vi "DAQ_daqmx.vi"() -> ()   [LabVIEW 2020]
uses:
  <vilib>/Utility/error.llb/DialogType.ctl
  <vilib>/Utility/sysdir.llb/System Directory Type.ctl
  <vilib>/DAQmx/read.llb/DAQmx Read (Analog 2D DBL NChan NSamp).vi
  <vilib>/DAQmx/create/channels.llb/DAQmx Create Channel (AI-Voltage-Basic).vi
  <vilib>/DAQmx/configure/timing.llb/DAQmx Timing (Sample Clock).vi
  <vilib>/DAQmx/configure/trigger.llb/DAQmx Start Trigger (None).vi
  <vilib>/DAQmx/miscellaneous.llb/DAQmx Fill In Error Info.vi
panel:
  in  "Save Button":bool
  out "Waveform Chart 2":dbl[][](graph)
  out "data":dbl[][](array[numeric]) format="%0.2f"
  in  "stop":bool
  out "Waveform Chart":dbl[][](graph)
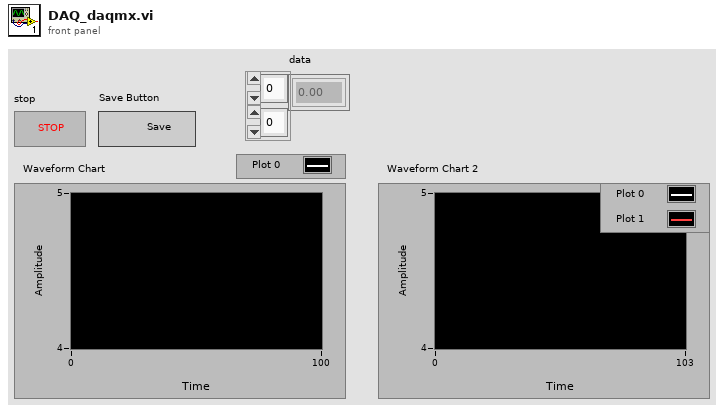
[diagram p1: front panel]
types:
  T1 = typedef "DialogType.ctl" = u16
  T2 = typedef "System Directory Type.ctl" = i32
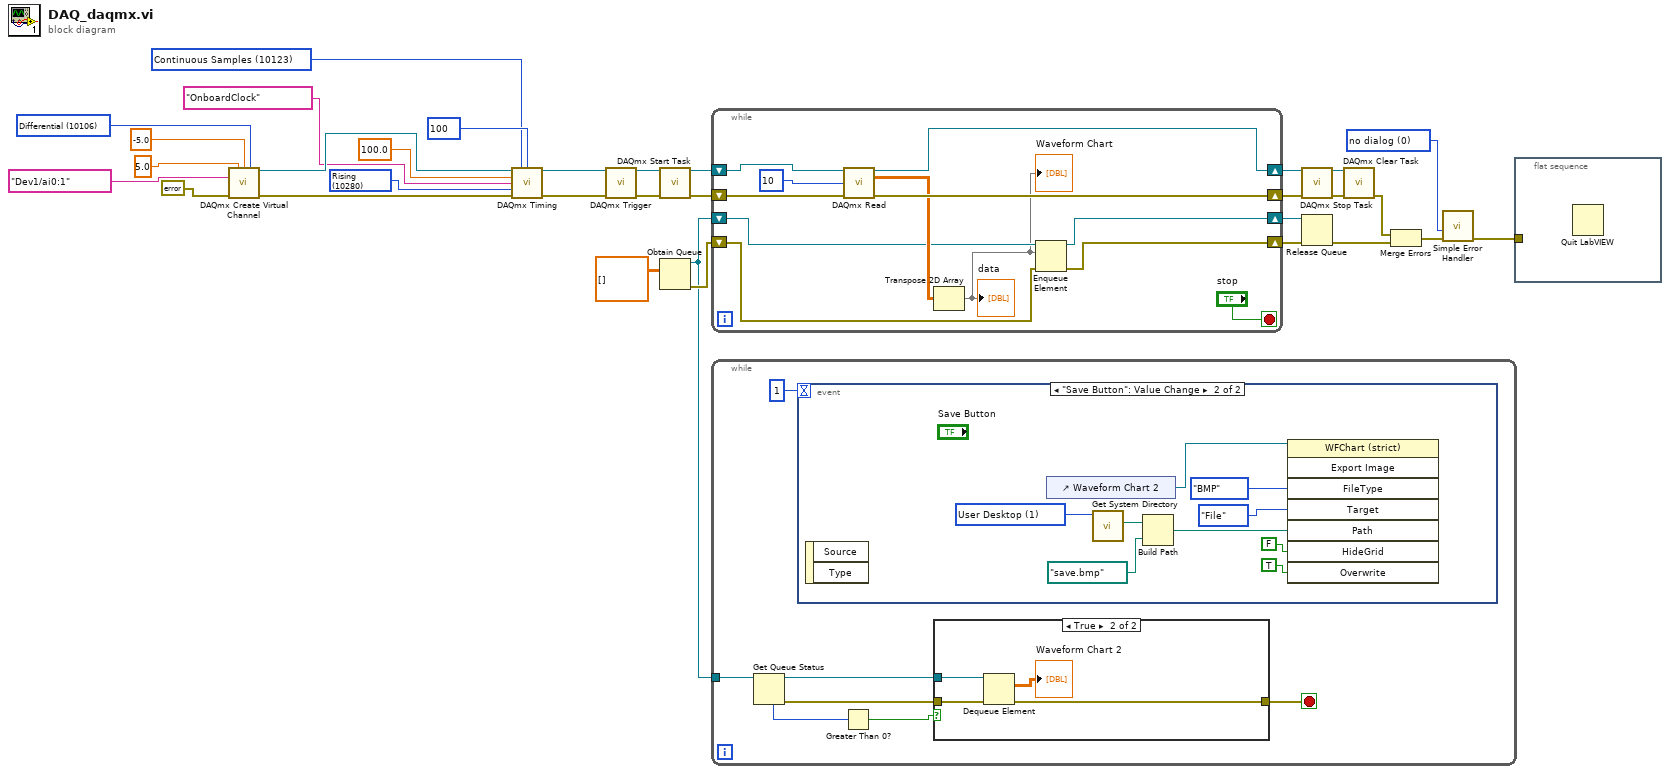
[diagram p0: block diagram]
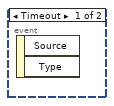
[diagram p2: hidden frame]
diagram:
  w10 = T1 0 items=["no dialog", "OK message", "continue or stop message", "OK message + warnings", "continue/stop + warnings"] ("type of dialog (OK msg:1)")
  w21 = 10280 items=["Rising"=10280, "Falling"=10171] ("active edge")
  w24 = 10123 items=["Finite Samples"=10178, "Continuous Samples"=10123, "Hardware Timed Single Point"=12522] ("sample mode")
  w32 = 10106 items=["Default"=-1, "RSE"=10083, "NRSE"=10078, "Differential"=10106, "Pseudodifferential"=12529] ("input terminal configuration")
  n1 = call-poly <vilib>:"DAQmx Create Virtual Channel.vi"("maximum value"=5.0, "minimum value"=-5.0, "input terminal configuration"=w32, "physical channels"=tag "Dev1/ai0:1", "error in"=errorcluster {"status"=FALSE, "code"=0, "source"=""}) -> ("task out"=w27:refnum<k21>, "error out"=w26:errorcluster)  [unwired: 9 in]
  n2 = call-poly <vilib>:"DAQmx Timing.vi"("task/channels in"=w27, "sample mode"=w24, "samples per channel"=100, "rate"=100.0, "source"=tag "OnboardClock", "active edge"=w21, "error in"=w26) -> ("task out"=w19:refnum<k21>, "error out"=w20:errorcluster)  [unwired: 7 in]
  n3 = call-poly <vilib>:"DAQmx Trigger.vi"("task/channels in"=w19, "error in"=w20) -> ("task out"=w18:refnum<k21>, "error out"=w17:errorcluster)  [unwired: 12 in]
  n4 = call <vilib>:"DAQmx Start Task.vi"("task/channels in"=w18, "error in"=w17) -> ("task out"=w16:refnum<k21>, "error out"=w15:errorcluster)  [unwired: 12 in]
  n5 = Obtain Queue(element data type=dbl[][] []) -> (queue out=w2:refnum<queue>, error out=w8:errorcluster)  [unwired: 4 in, 1 out]
  n6 = while {
    shift-right: [w42] -> w14
    shift-left: w16 -> [w44]
    shift-right: [w41] -> w13
    shift-left: w15 -> [w43]
    shift-right: [w34] -> w7
    shift-left: w2 -> [w37]
    shift-right: [w33] -> w6
    shift-left: w8 -> [w36]
    stop <- "stop" stop-if-true
    n7 = call-poly <vilib>:"DAQmx Read.vi"("task/channels in"=w44, "number of samples per channel"=10, "error in"=w43) -> ("task out"=w42:refnum<k21>, "data"=w39:dbl[][], "error out"=w41:errorcluster)  [unwired: 10 in]
    n8 = Transpose 2D Array(2D array=w39) -> (transposed array=w35:dbl[][])
    "Waveform Chart" <- w35
    "data" <- w35
    n9 = Enqueue Element(queue=w37, element=w35, error in (no error)=w36) -> (queue out=w34:refnum<queue>, error out=w33:errorcluster)  [unwired: 1 in, 1 out]
  }
  n10 = while {
    tunnel: w2 -> [w51]
    stop <- w47 stop-if-true
    n11 = Get Queue Status(queue=w51) -> (queue out=w49:refnum<queue>, error out=w48:errorcluster, # elements in queue=w50:i32)  [unwired: 2 in, 5 out]
    n12 = event shown="[1] \"Save Button\": Value Change" {
      selector: _ -> [_ _]
      dyn-events: _ -> [_ _]
      timeout: 1 -> [_ _]
      event Timeout {
        n13 = event-data() -> ()  [unwired: 1 in, 2 out]
      }
      event "Save Button": Value Change {
        w56 = T2 1 items=["User Home"=0, "User Desktop"=1, "User Documents"=2, "User Application Data"=3, "User Preferences"=4, "User Temporary"=5, "Public Documents"=6, "Public Application Data"=7, "Public Preferences"=8, "Public Cache"=13, "System Core Libraries"=9, "System Installed Libraries"=10, "Application Files"=11, "Boot Volume Root"=12] ("system directory type")
        n14 = event-data() -> ()  [unwired: 1 in, 2 out]
        n15 = control-ref of="Waveform Chart 2"() -> (w52:refnum<vi>)
        n16 = call <vilib>:"Get System Directory.vi"("system directory type"=w56) -> ("system directory"=w55:path)  [unwired: 10 in]
        n17 = Build Path(base path=w55, name or relative path=path "save.bmp") -> (appended path=w53:path)
        n18 = invoke class="WFChart (strict)" method="Export Image"(reference=w52, "FileType"=enum32{"BMP", "EPS", "EMF", "PICT"}."BMP" ("File Type"), "Target"=enum32{"File", "Clipboard"}."File", "Path"=w53, "HideGrid"=FALSE ("Hide Grid"), "Overwrite"=TRUE ("Always Overwrite")) -> ()  [unwired: 2 in, 8 out]
      }
    }
    n19 = Greater Than 0?(x=w50) -> (x > 0?=w46:bool)
    n20 = case shown="True" w46 {
      tunnel: w49 -> [_ w65]
      tunnel: w48 -> [w61 w64]
      tunnel: [w61 w62] -> w47
      frame False {
      }
      frame True {
        n21 = Dequeue Element(queue=w65, error in (no error)=w64) -> (element=→"Waveform Chart 2":dbl[][], error out=w62:errorcluster)  [unwired: 1 in, 2 out]
      }
    }
  }
  n22 = call <vilib>:"DAQmx Stop Task.vi"("task/channels in"=w14, "error in"=w13) -> ("task out"=w12:refnum<k21>, "error out"=w11:errorcluster)  [unwired: 12 in]
  n23 = Release Queue(queue=w7, error in (no error)=w6) -> (error out=w4:errorcluster)  [unwired: 1 in, 2 out]
  n24 = call <vilib>:"DAQmx Clear Task.vi"("task in"=w12, "error in"=w11) -> ("error out"=w5:errorcluster)  [unwired: 13 in]
  n25 = Merge Errors(w5, w4) -> (w3:errorcluster)
  n26 = call <vilib>:"Simple Error Handler.vi"("type of dialog (OK msg:1)"=w10, "error in (no error)"=w3) -> ("error out"=w1:errorcluster)  [unwired: 3 in, 4 out]
  n27 = flat-sequence {
    tunnel: w1 -> [_]
    frame #0 {
      n28 = Quit LabVIEW() -> ()  [unwired: 1 in]
    }
  }
